vi "Draw.vi"(7 "Packed refs":T1, 8 "error in (no error)":errorcluster, 10 "This VI":refnum<vi>, 11 "Board Game in":refnum<class "Board Game.lvclass">) -> (0 "error out":errorcluster, 3 "Board Game out":refnum<class "Board Game.lvclass">)   [LabVIEW 2021, in "Board Game.lvclass"]
uses:
  Board Game.lvclass
  Application/Packed Refs.ctl
  GameEl_class/private/Enum Direction.ctl
  Board Game.lvclass/Board Game.ctl
  Snake_class/Snake.lvclass/Snake.ctl
  Snake_class/Read Bomb Crash.vi
  <userlib>/_OpenG.lib/comparison/comparison.llb/Variant Changed__ogtk.vi
  Snake_class/Snake.lvclass
  <userlib>/_OpenG.lib/comparison/comparison.llb/openg_comparison__ogtk.lvlib
  GameEl_class/GameEl.lvclass
  Application/Game.lvclass
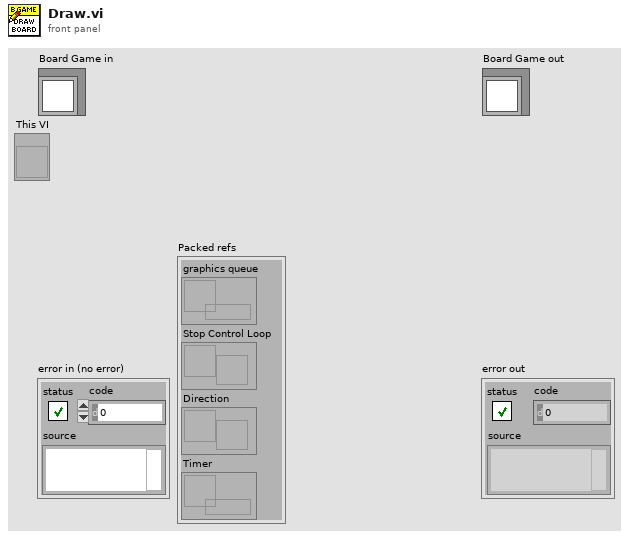
[diagram p1: front panel]
types:
  T1 = typedef "Game.lvclass/Packed Refs.ctl" = cluster{"graphics queue":refnum<queue>, "Stop Control Loop":refnum<user-event>, "Direction":refnum<notifier>, "Timer":refnum<data-value>}
  T2 = cluster{"Colour":u32, "position":cluster{"x":dbl, "y":dbl}}[]
  T3 = cluster{"Snake":refnum<class "Snake.lvclass">, "Board Game in":refnum<class "Board Game.lvclass">}
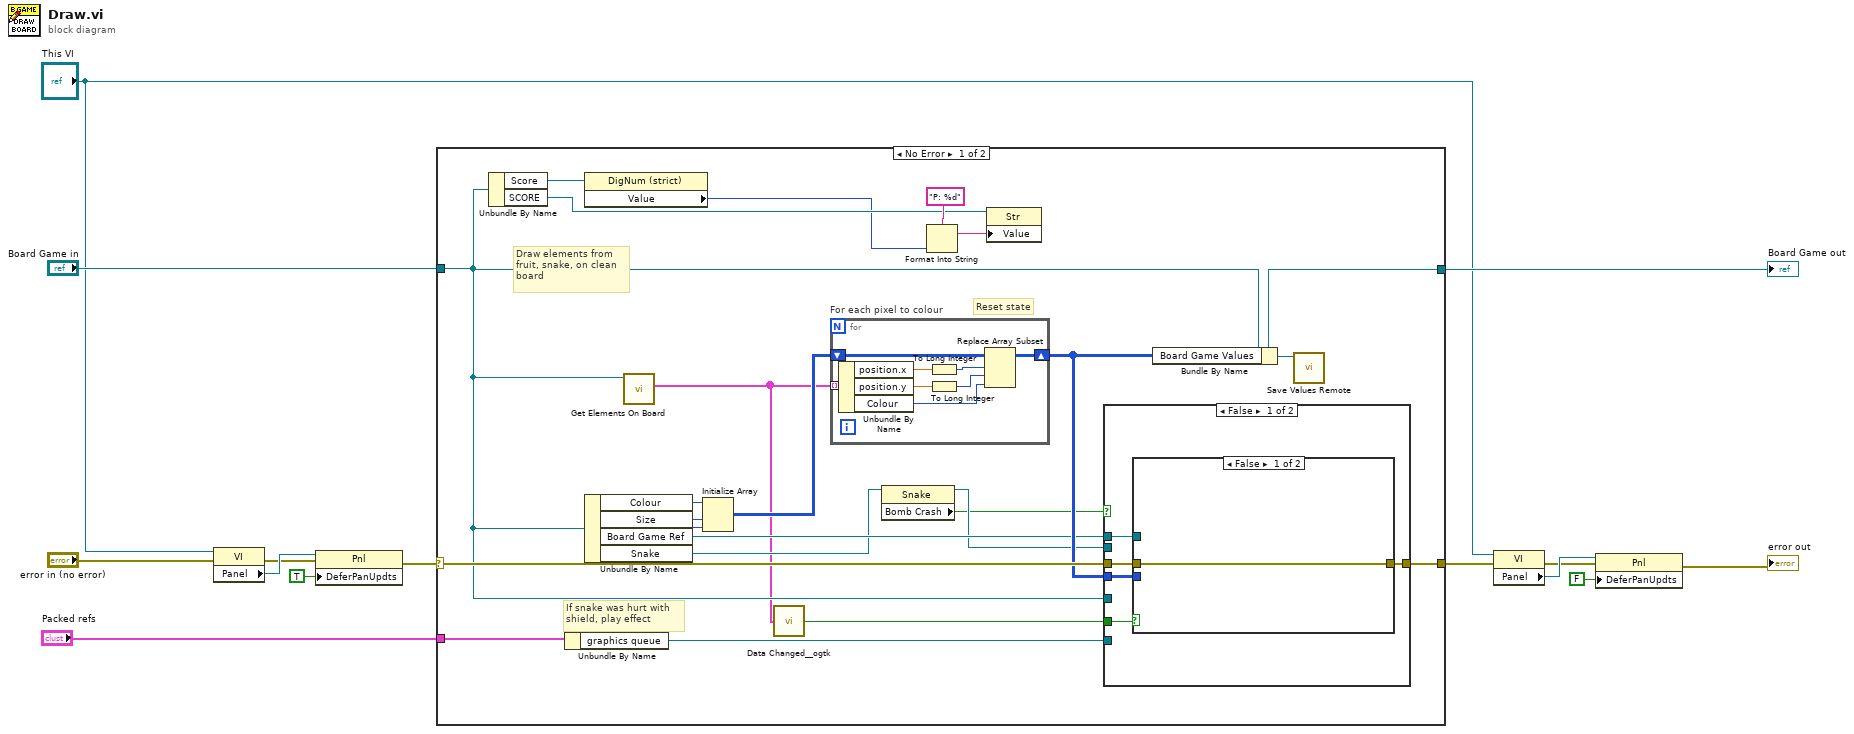
[diagram p0: block diagram]
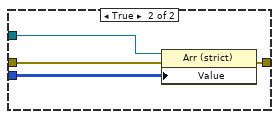
[diagram p2: hidden frame]
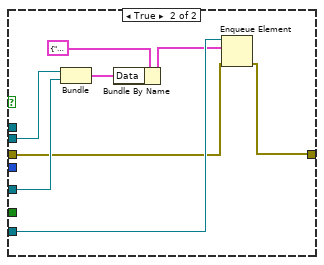
[diagram p3: hidden frame]
diagram:
  n1 = property class="VI"(reference="This VI", error in="error in (no error)") -> (error out=w8:errorcluster, "Panel"=w10:refnum<vi>)  [unwired: 1 out]
  n2 = property class="Pnl"(reference=w10, error in=w8, "DeferPanUpdts"=TRUE ("Defer Panel Updates")) -> (error out=w7:errorcluster)  [unwired: 1 out]
  n3 = case shown="No Error" w7 {
    selector: w7 -> [w35 w63]
    tunnel: [w33 w63] -> w3
    tunnel: [w26 w62] -> w13
    tunnel: "Board Game in" -> [w23 w62]
    tunnel: "Packed refs" -> [w28 _]
    frame No Error {
      # "Reset state"
      # "If snake was hurt with \nshield, play effect"
      # "Draw elements from \nfruit, snake, on clean \nboard"
      n4 = Unbundle By Name(w23) -> ("Score"=w22:refnum<vi>, "SCORE"=w21:refnum<vi>)
      n5 = Unbundle By Name(w28) -> ("graphics queue"=w27:refnum<queue>)
      n6 = property class="DigNum (strict)"(reference=w22) -> ("Value"=w20:u16)  [unwired: 1 in, 2 out]
      n7 = Unbundle By Name(w23) -> ("Colour"=w29:u32, "Size"=w32:u16, "Board Game Ref"=w30:refnum<vi>, "Snake"=w19:refnum<class "Snake.lvclass">)
      n8 = call "Get Elements On Board.vi"("Board Game in"=w23) -> ("Color Array"=w16:T2)  [unwired: 9 in, 1 out]
      n9 = Initialize Array(w29, w32, w32) -> (w31:u32[][])
      n10 = call-poly <userlib>:"Data Changed__ogtk.vi"("Variant"=w16) -> ("Changed"=w15:bool)
      n11 = for "For each pixel to colour" {
        shift-right: [w59] -> w34
        shift-left: w31 -> [w60]
        tunnel: w16 -> [w61] mode=indexing
        n12 = Unbundle By Name(w61) -> ("position.x"=w58:dbl, "position.y"=w57:dbl, "Colour"=w56:u32)
        n13 = To Long Integer(number=w58) -> (32bit integer=w55:i32)
        n14 = To Long Integer(number=w57) -> (32bit integer=w54:i32)
        n15 = Replace Array Subset(array=w60, new element=w56, index (row)=w55, index (col)=w54) -> (w59:u32[][])
      }
      n16 = property class="Snake"(reference=w19) -> (reference out=w18:refnum<class "Snake.lvclass">, "Bomb Crash"=w17:bool)  [unwired: 1 in, 1 out]
      n17 = Format Into String(format string="P: %d", w20) -> (resulting string=w25:string)  [unwired: 2 in, 1 out]
      n18 = property class="Str"(reference=w21, "Value"=w25) -> ()  [unwired: 1 in, 2 out]
      n19 = case shown="False" w17 {
        tunnel: w35 -> [w40 w47]
        tunnel: w34 -> [w39 _]
        tunnel: [w38 w46] -> w33
        tunnel: w30 -> [w37 _]
        tunnel: w18 -> [_ w53]
        tunnel: w23 -> [_ w52]
        tunnel: w27 -> [_ w51]
        tunnel: w15 -> [w36 _]
        frame False {
          n20 = case shown="False" w36 {
            tunnel: w40 -> [w41 w45]
            tunnel: w39 -> [_ w44]
            tunnel: [w41 w43] -> w38
            tunnel: w37 -> [_ w42]
            frame False {
            }
            frame True {
              n21 = property class="Arr (strict)"(reference=w42, error in=w45, "Value"=w44) -> (error out=w43:errorcluster)  [unwired: 1 out]
            }
          }
        }
        frame True {
          n22 = Bundle("Snake"=w53, "Board Game in"=w52) -> (w49:T3)  [unwired: 1 in]
          n23 = Bundle By Name(cluster=cluster{"Message":string, "Data":variant} {"Message"="Blink Game Element", "Data"=variant} ("element"), "Data"=w49) -> (w48:cluster{"Message":string, "Data":variant})
          n24 = Enqueue Element(queue=w51, element=w48, error in (no error)=w47) -> (error out=w46:errorcluster)  [unwired: 1 in, 2 out]
        }
      }
      n25 = Bundle By Name(cluster=w23, "Board Game Values"=w34) -> (w26:refnum<class "Board Game.lvclass">)
      n26 = call "Save Values Remote.vi"("Board Game in"=w26) -> ()  [unwired: 10 in, 1 out]
    }
    frame Error {
    }
  }
  "Board Game out" <- w13
  n27 = property class="VI"(reference="This VI", error in=w3) -> (error out=w4:errorcluster, "Panel"=w6:refnum<vi>)  [unwired: 1 out]
  n28 = property class="Pnl"(reference=w6, error in=w4, "DeferPanUpdts"=FALSE ("Defer Panel Updates")) -> (error out=→"error out":errorcluster)  [unwired: 1 out]
